vi "Get Analog DataSet MultiRow & ChanNames DataQ.vi"(6 "QueueName String (optional, otherwise \"\")":variant, 8 "error in (no error)":errorcluster, 9 "Select":T2, 10 "TaskName":string, 11 "DataQueues in":refnum<class "DataQueues.lvclass">) -> (0 "error out":errorcluster, 1 "Analog DataSet MultiRow & ChanNames QRef":T1, 2 "TaskName out":string, 3 "DataQueues out":refnum<class "DataQueues.lvclass">, 4 "QueueName":string)   [LabVIEW 2017, in "DataQueues.lvclass"]
doc: "Developed by Kevin Thompson\nkevin@thompsonengineering.net\n\nCopyright 2018-2020\nThompson Engineering, LLC"
uses:
  DataQueues.lvclass
  DataTypes/DataQ SelectType--enum.ctl
  DataTypes/Analog DataSet MultiRow & ChanNames--QRef.ctl
  DataTypes/Analog DataSet MultiRow & ChanNames--cluster.ctl
  DataQueues.lvclass/DataQueues.ctl
  DataTypes/DataQ Ref DictNode--cluster.ctl
  Accessors/Get DataQ Dict.vi
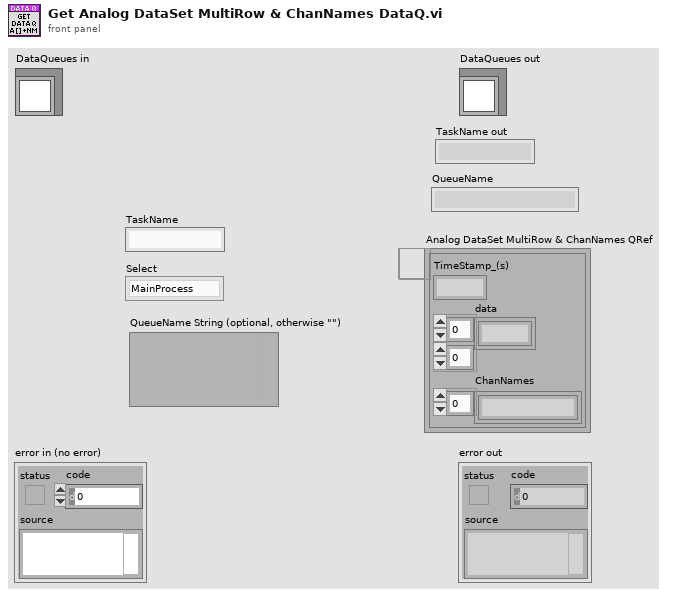
[diagram p1: front panel]
types:
  T1 = typedef "DataQueues.lvclass/Analog DataSet MultiRow & ChanNames--QRef.ctl" = refnum<queue>
  T2 = typedef "DataQueues.lvclass/DataQ SelectType--enum.ctl" = enum16{"MainProcess", "LogEngine", "LocalDAQThread"}
  T3 = typedef "DataQueues.lvclass/DataQ Ref DictNode--cluster.ctl" = cluster{"KeyName":string, "Type Name":string, "vDataQ Ref":variant}
  T4 = typedef "TD Dynamic CVT DVR--ref.ctl" = refnum<data-value>
  T5 = typedef "Type Descriptor Enumeration__ogtk.ctl" = enum8{"<Null>", "I8", "I16", "I32", "I64", "U8", "U16", "U32", "U64", "SGL", "DBL", "EXT", "CSG", "CDB", "CXT", "0x0F", "0x10", "0x11", "0x12", "0x13", "0x14", "Enum U8", "Enum U16", "Enum U32", "Enum U64", "SGL PQ", "DBL PQ", "EXT PQ", "CSG PQ", "CDB PQ", "CXT PQ", "0x1F", "0x20", "Boolean", "0x22", "0x23", "0x24", "0x25", "0x26", "0x27", "0x28", "0x29", "0x2A", "0x2B", "0x2C", "0x2D", "0x2E", "0x2F", "String", "0x31", "Path", "Pict", "0x34", "0x35", "0x36", "DAQ", "0x38", "0x39", "0x3A", "0x3B", "0x3C", "0x3D", "0x3E", "0x3F", "Array", "0x41", "0x42", "0x43", "0x44", "0x45", "0x46", "0x47", "0x48", "0x49", "0x4A", "0x4B", "0x4C", "0x4D", "0x4E", "0x4F", "Cluster", "0x51", "0x52", "Variant", "Waveform", "0x55", "0x56", "0x57", "0x58", "0x59", "0x5A", "0x5B", "0x5C", "0x5D", "0x5E", "0x5F", "0x60", "0x61", "0x62", "0x63", "0x64", "0x65", "0x66", "0x67", "0x68", "0x69", "0x6A", "0x6B", "0x6C", "0x6D", "0x6E", "0x6F", "Refnum"}
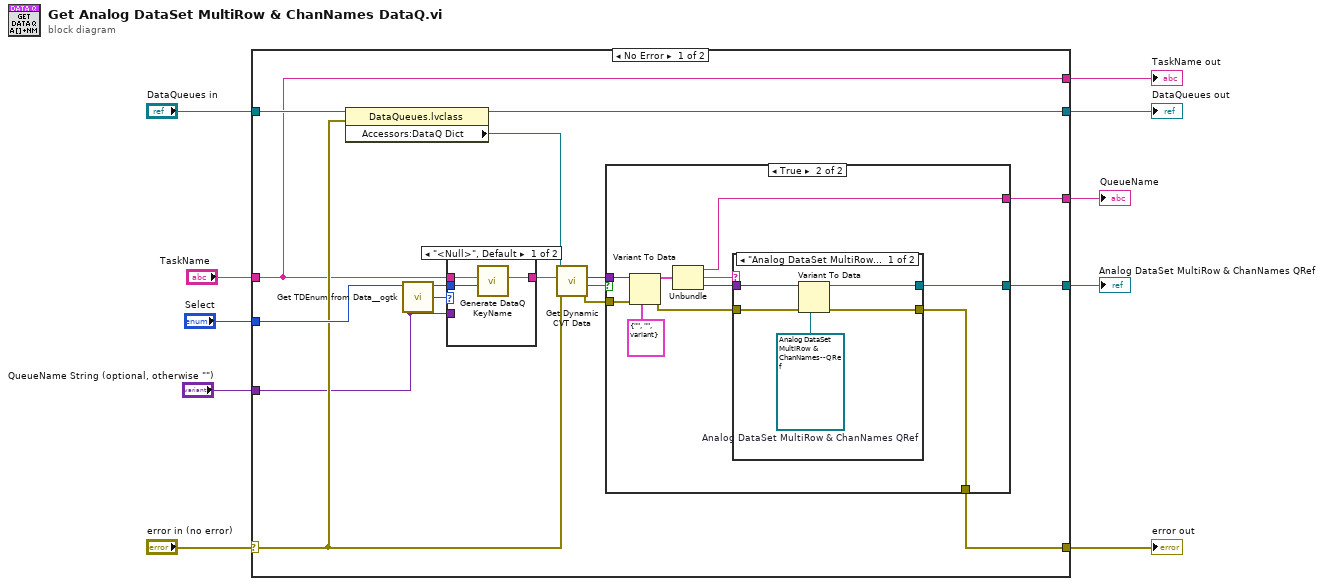
[diagram p0: block diagram]
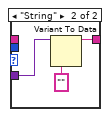
[diagram p2: hidden frame]
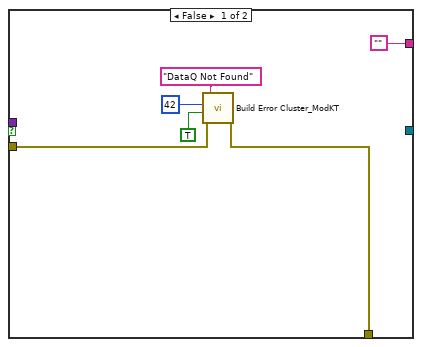
[diagram p3: hidden frame]
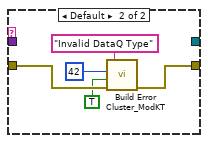
[diagram p4: hidden frame]
diagram:
  n1 = case shown="No Error" "error in (no error)" {
    selector: "error in (no error)" -> [w21 w60]
    tunnel: [w23 w60] -> w9
    tunnel: [w14 w59] -> w7
    tunnel: "DataQueues in" -> [w24 w59]
    tunnel: "TaskName" -> [w11 w58]
    tunnel: "Select" -> [w25 _]
    tunnel: "QueueName String (optional, otherwise \"\")" -> [w15 _]
    tunnel: [w13 _] -> w2
    tunnel: [w12 _] -> w3
    tunnel: [w11 w58] -> w1
    frame No Error {
      n2 = property class="DataQueues.lvclass"(reference=w24, error in=w21) -> (reference out=w14:refnum<class "DataQueues.lvclass">, "Accessors:DataQ Dict"=w22:T4)  [unwired: 1 out]
      n3 = call <userlib>:"Get TDEnum from Data__ogtk.vi"("Data"=w15) -> ("Type Descriptor Enumeration"=w16:T5)  [unwired: 4 in]
      n4 = case shown="\"<Null>\", Default" w16 {
        tunnel: w11 -> [w28 _]
        tunnel: w25 -> [w27 _]
        tunnel: [w26 w31] -> w20
        tunnel: w15 -> [_ w30]
        frame "<Null>", Default {
          n5 = call "Generate DataQ KeyName.vi"("Select"=w27, "TaskName"=w28) -> ("DataQ KeyName"=w26:string)  [unwired: 9 in]
        }
        frame "String" {
          n6 = Variant To Data(type="", Variant=w30) -> (data=w31:string)  [unwired: 1 in, 1 out]
        }
      }
      n7 = call <vilib>:"Get Dynamic CVT Data.vi"("error in (no error)"=w21, "DataName"=w20, "dCVT DVR"=w22) -> ("error out"=w18:errorcluster, "found"=w17:bool, "value"=w19:variant)  [unwired: 5 in, 1 out]
      n8 = case shown="True" w17 {
        tunnel: [w33 w39] -> w23
        tunnel: w19 -> [_ w47]
        tunnel: w18 -> [w34 w46]
        tunnel: ["" w40] -> w12
        tunnel: [_ w38] -> w13
        frame False {
          n9 = call <vilib>:"Build Error Cluster_ModKT .vi"("Prepend String (\"\")"="DataQ Not Found" ("Prepend String (\"\")"), "code"=42, "error? (F)"=TRUE, "error in (no error)"=w34) -> ("error out"=w33:errorcluster)  [unwired: 3 in, 1 out]
        }
        frame True {
          n10 = Variant To Data(error in=w46, type=T3 {"KeyName"="", "Type Name"="", "vDataQ Ref"=variant} ("DataQ Ref DictNode"), Variant=w47) -> (data=w44:T3, error out=w42:errorcluster)
          n11 = Unbundle(w44) -> ("KeyName"=w40:string, "Type Name"=w41:string, "vDataQ Ref"=w43:variant)
          n12 = case shown="\"Analog DataSet MultiRow & ChanNames\"" w41 {
            tunnel: w43 -> [w52 _]
            tunnel: w42 -> [w50 w57]
            tunnel: [w48 w56] -> w39
            tunnel: [w49 _] -> w38
            frame "Analog DataSet MultiRow & ChanNames" {
              w51 = T1 refnum  # Analog DataSet MultiRow & ChanNames QRef
              n13 = Variant To Data(error in=w50, type=w51, Variant=w52) -> (data=w49:T1, error out=w48:errorcluster)
            }
            frame Default {
              n14 = call <vilib>:"Build Error Cluster_ModKT .vi"("Prepend String (\"\")"="Invalid DataQ Type" ("Prepend String (\"\")"), "code"=42, "error? (F)"=TRUE, "error in (no error)"=w57) -> ("error out"=w56:errorcluster)  [unwired: 3 in, 1 out]
            }
          }
        }
      }
    }
    frame Error {
    }
  }
  "error out" <- w9
  "DataQueues out" <- w7
  "QueueName" <- w3
  "Analog DataSet MultiRow & ChanNames QRef" <- w2
  "TaskName out" <- w1
